vi "MeasureSystemOffset.vi"(8 "error in":errorcluster, 10 "Number of averages":u32=1, 11 "VISA resource name":refnum<visa-resource-name>) -> (0 "error out":errorcluster, 2 "Device offset from local / us":ext format="%.3f", 3 "VISA resource name out":refnum<visa-resource-name>)   [LabVIEW 2018, in "GP22_TDC_Arduinoed.lvlib"]
doc: "Use a basic version of NTP to calculate the offset of the device's system clock from the local PC's system clock."
uses:
  GP22_TDC_Arduinoed.lvlib
panel:
  out "Offset / us":ext(graph)
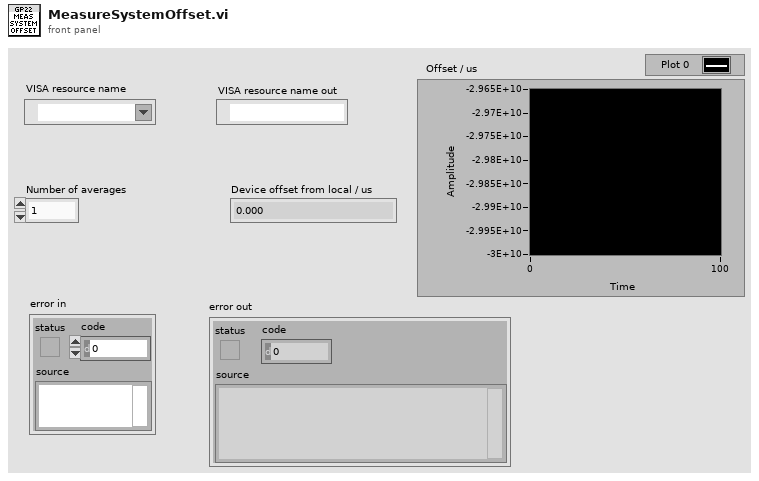
[diagram p1: front panel]
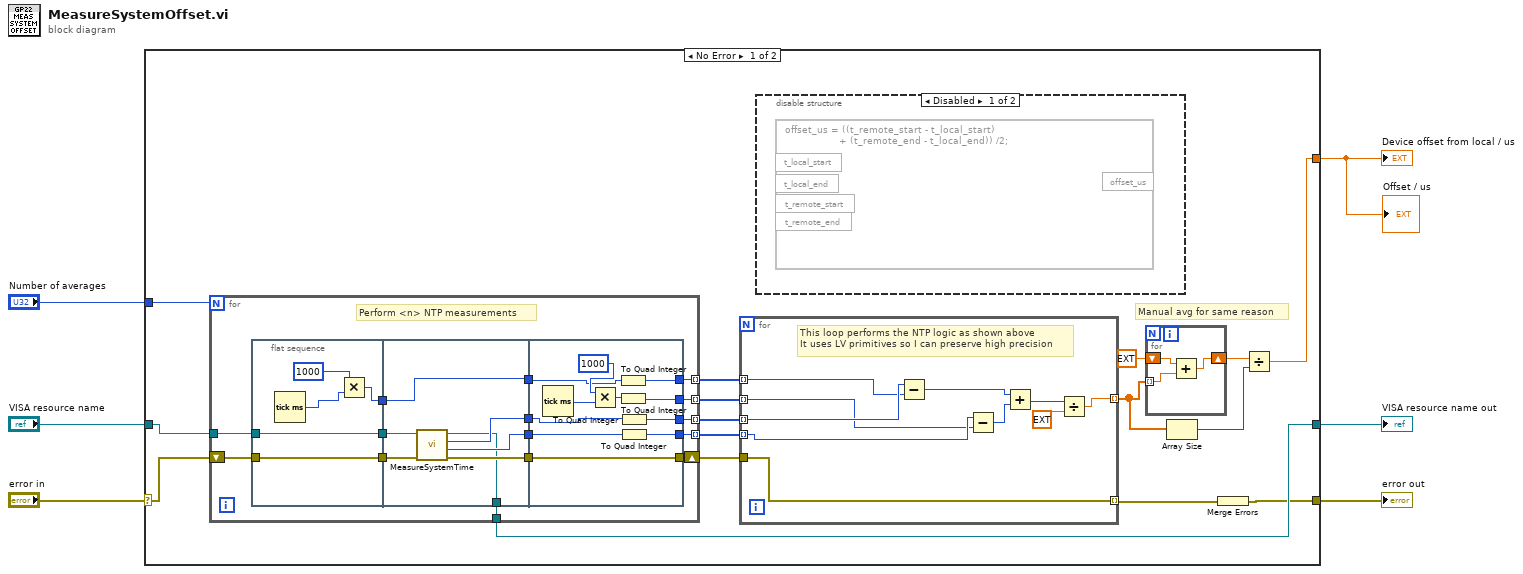
[diagram p0: block diagram]
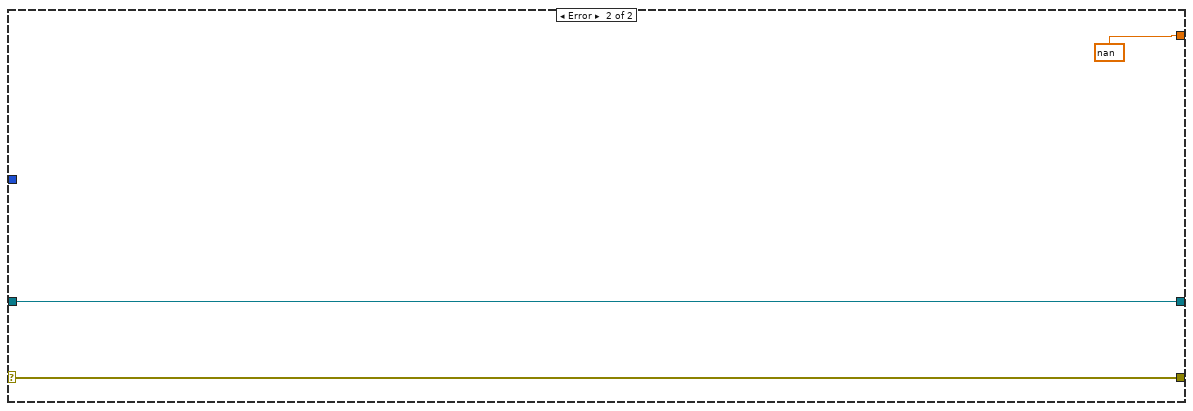
[diagram p3: hidden frame]
diagram:
  n1 = case shown="No Error" "error in" {
    selector: "error in" -> [w21 w76]
    tunnel: [w15 w75] -> w6
    tunnel: "VISA resource name" -> [w22 w75]
    tunnel: [w14 w76] -> w3
    tunnel: "Number of averages" -> [w20 _]
    tunnel: [w7 nan] -> w1
    frame No Error {
      # "Manual avg for same reason"
      n2 = for {
        N: w20 -> [_]
        tunnel: w22 -> [w50]
        shift-right: [w48] -> w19
        shift-left: w21 -> [w49]
        tunnel: [w47] -> w16 mode=indexing
        tunnel: [w39] -> w18 mode=indexing
        tunnel: [w38] -> w17 mode=indexing
        tunnel: [w37] -> w15
        tunnel: [w36] -> w12 mode=indexing
        # "Perform <n> NTP measurements"
        n3 = flat-sequence {
          tunnel: w49 -> [w54]
          tunnel: w50 -> [w55]
          tunnel: [w55] -> w46
          tunnel: [w54] -> w45
          tunnel: [w52] -> w44
          tunnel: w46 -> [w62]
          tunnel: w45 -> [w61]
          tunnel: w44 -> [w57]
          tunnel: [w60] -> w43
          tunnel: [w59] -> w42
          tunnel: [w58] -> w41
          tunnel: [w57] -> w40
          tunnel: [w56] -> w37
          tunnel: [w66] -> w39
          tunnel: [w68] -> w47
          tunnel: [w73] -> w48
          tunnel: w43 -> [w73]
          tunnel: w42 -> [w69]
          tunnel: w41 -> [w67]
          tunnel: w40 -> [w63]
          tunnel: [w65] -> w38
          tunnel: [w70] -> w36
          frame #0 {
            n4 = Tick Count (ms)() -> (millisecond timer value=w53:u32)
            n5 = Multiply(x=u64 1000, y=w53) -> (x*y=w52:u64)
          }
          frame #1 {
            n6 = call "MeasureSystemTime.vi"("error in"=w61, "VISA resource name"=w62) -> ("error out"=w60:errorcluster, "System time end / us"=w58:u32, "System time start / us"=w59:u32, "VISA resource name out"=w56:refnum<visa-resource-name>)  [unwired: 6 in]
          }
          frame #2 {
            n7 = Tick Count (ms)() -> (millisecond timer value=w71:u32)
            n8 = Multiply(x=u64 1000, y=w71) -> (x*y=w64:u64)
            n9 = To Quad Integer(1:w63) -> (0:w66:i64)
            n10 = To Quad Integer(1:w64) -> (0:w65:i64)
            n11 = To Quad Integer(1:w69) -> (0:w70:i64)
            n12 = To Quad Integer(1:w67) -> (0:w68:i64)
          }
        }
      }
      n13 = for {
        tunnel: w19 -> [w35]
        tunnel: w18 -> [w33] mode=indexing
        tunnel: w17 -> [w31] mode=indexing
        tunnel: w16 -> [w32] mode=indexing
        tunnel: [w35] -> w13 mode=indexing
        tunnel: [w26] -> w8 mode=indexing
        tunnel: w12 -> [w34] mode=indexing
        # "This loop performs the NTP logic as shown above\nIt uses LV primitives so I can preserve high precision"
        n14 = Subtract(x=w34, y=w33) -> (x-y=w29:i64)
        n15 = Subtract(x=w32, y=w31) -> (x-y=w30:i64)
        n16 = Add(x=w29, y=w30) -> (x+y=w28:i64)
        n17 = Divide(x=w28, y=ext 2.0) -> (x/y=w26:ext)
      }
      n18 = disable-structure shown="Disabled" {
        frame Disabled {
          n19 = formula code="offset_us = ((t_remote_start - t_local_start) \n                  + (t_remote_end - t_local_end)) /2;"() -> ()  [unwired: 4 in, 1 out]
        }
        frame Enabled {
        }
      }
      n20 = for {
        tunnel: w8 -> [w24] mode=indexing
        shift-right: [w23] -> w10
        shift-left: ext 0.0 -> [w25]
        n21 = Add(x=w25, y=w24) -> (x+y=w23:ext)
      }
      n22 = Array Size(array=w8) -> (size(s)=w9:i32)
      n23 = Merge Errors(w13) -> (w14:errorcluster)
      n24 = Divide(x=w10, y=w9) -> (x/y=w7:ext)
    }
    frame Error {
    }
  }
  "VISA resource name out" <- w6
  "error out" <- w3
  "Device offset from local / us" <- w1
  "Offset / us" <- w1
